vi "Get PID Values.vi"() -> (0 "PID gains Out":T1={"proportional gain (Kc)"=0.0111, "integral time (Ti, min)"=0.007, "derivative time (Td, min)"=0.0})   [LabVIEW 2011, in "Pivot Drive.lvlib"]
doc: "Gets the PID values that are being used by the pivot system.\nBy default the constants are:\nKc=.0111\nI=.007\nD=0\nThese are the values that worked for team 1640."
uses:
  Pivot Drive.lvlib
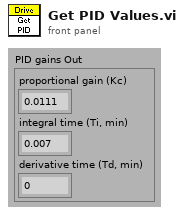
[diagram p1: front panel]
types:
  T1 = cluster{"proportional gain (Kc)":dbl, "integral time (Ti, min)":dbl, "derivative time (Td, min)":dbl}
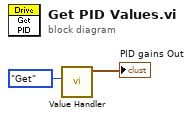
[diagram p0: block diagram]
diagram:
  n1 = call "Value Handler.vi"("Set or Get"=enum16{"Set", "Get"}."Get") -> ("PID gains Out"=→"PID gains Out":T1)  [unwired: 1 in, 9 out]
